vi "baratron_conv_analog.vi"(10 "V_ana (V)":dbl) -> (2 "y (Pa)":dbl)   [LabVIEW 2017]
uses:
  <vilib>/express/express arith-compare/Formula/XNode/ExpressFormulaBlockNode.xnode
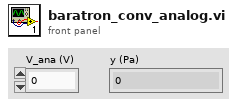
[diagram p1: front panel]
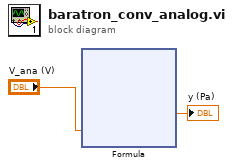
[diagram p0: block diagram]
diagram:
  n1 = xnode "Formula"("X"="V_ana (V)") -> ("結果"=→"y (Pa)":dbl)  [unwired: 1 in, 1 out]
